vi "M Water Cells.vi"(11 "EV3 in":T1) -> (3 "EV3 out":T1)   [LabVIEW 2016]
uses:
  <vilib>/NXT/Subs/LVHSConnector.ctl
  <vilib>/NXT/LegoClasses/BrickReference/BrickReference.lvclass
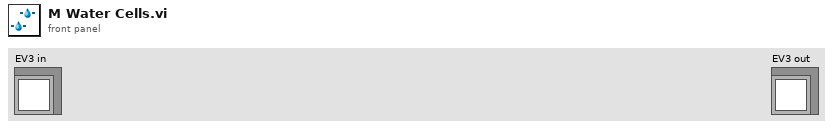
[diagram p1: front panel]
types:
  T1 = typedef "LVHSConnector.ctl" = refnum<class "BrickReference.lvclass">
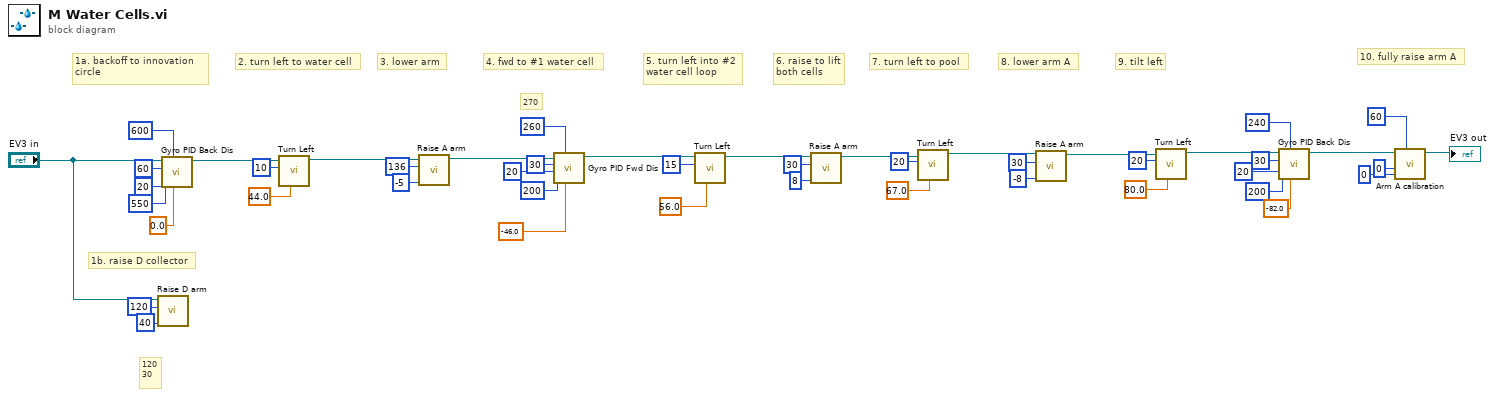
[diagram p0: block diagram]
diagram:
  # "270"
  # "120\n30"
  # "10. fully raise arm A"
  # "9. tilt left"
  # "8. lower arm A"
  # "7. turn left to pool"
  # "6. raise to lift\nboth cells"
  # "5. turn left into #2\nwater cell loop"
  # "4. fwd to #1 water cell"
  # "3. lower arm"
  # "2. turn left to water cell"
  # "1b. raise D collector"
  # "1a. backoff to innovation\ncircle"
  n1 = call "Raise D arm.vi"("Power"=i8 40, "Rotation"=120, "EV3 in"="EV3 in") -> ()  [unwired: 8 in, 1 out]
  n2 = call "Gyro PID Back Dis.vi"("Target angle"=sgl 0.0, "Threshold to stop"=600, "Threshold to slow"=550, "Min. speed"=20, "Max. speed"=60, "EV3 in"="EV3 in") -> ("EV3 out"=w39:T1)  [unwired: 5 in]
  n3 = call "Turn Left.vi"("Turning angle"=sgl 44.0, "Motor B (right)"=i8 10, "EV3 in"=w39) -> ("EV3 out"=w36:T1)  [unwired: 8 in]
  n4 = call "Raise A arm.vi"("Power"=i8 -5, "Rotation"=136, "EV3 in"=w36) -> ("EV3 out"=w32:T1)  [unwired: 8 in]
  n5 = call "Gyro PID Fwd Dis.vi"("Target angle"=sgl -46.0, "Threshold to stop"=260, "Threshold to slow"=200, "Min. speed"=20, "Max. speed"=30, "EV3 in"=w32) -> ("EV3 out"=w26:T1)  [unwired: 5 in]
  n6 = call "Turn Left.vi"("Turning angle"=sgl 56.0, "Motor B (right)"=i8 15, "EV3 in"=w26) -> ("EV3 out"=w23:T1)  [unwired: 8 in]
  n7 = call "Raise A arm.vi"("Power"=i8 8, "Rotation"=30, "EV3 in"=w23) -> ("EV3 out"=w20:T1)  [unwired: 8 in]
  n8 = call "Turn Left.vi"("Turning angle"=sgl 67.0, "Motor B (right)"=i8 20, "EV3 in"=w20) -> ("EV3 out"=w17:T1)  [unwired: 8 in]
  n9 = call "Raise A arm.vi"("Power"=i8 -8, "Rotation"=30, "EV3 in"=w17) -> ("EV3 out"=w13:T1)  [unwired: 8 in]
  n10 = call "Turn Left.vi"("Turning angle"=sgl 80.0, "Motor B (right)"=i8 20, "EV3 in"=w13) -> ("EV3 out"=w11:T1)  [unwired: 8 in]
  n11 = call "Gyro PID Back Dis.vi"("Target angle"=sgl -82.0, "Threshold to stop"=240, "Threshold to slow"=200, "Min. speed"=20, "Max. speed"=30, "EV3 in"=w11) -> ("EV3 out"=w5:T1)  [unwired: 5 in]
  n12 = call "Arm A calibration.vi"("Cali. Power"=i8 60, "Down Power"=i8 0, "Rotation"=0, "NXT/EV3"=w5) -> ("NXT/EV3"=→"EV3 out":T1)  [unwired: 7 in]
